vi "Make_PS_Req.vi"(8 "error in (no error)":errorcluster, 11 "Request in":refnum<class "Request.lvclass">) -> (0 "error out":errorcluster, 1 "standard error":string, 2 "standard output":string, 3 "Request out":refnum<class "Request.lvclass">)   [LabVIEW 2016, in "Request.lvclass"]
uses:
  Request.lvclass
  Request.lvclass/Request.ctl
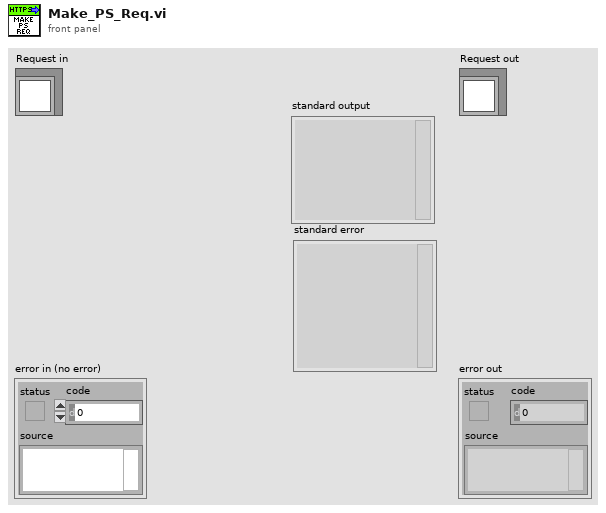
[diagram p1: front panel]
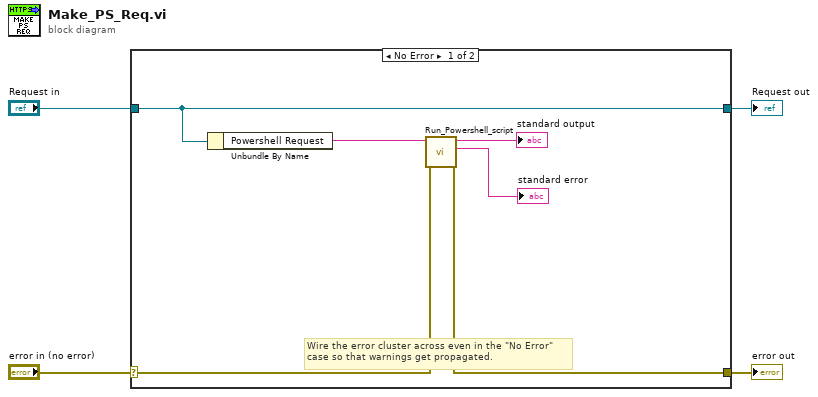
[diagram p0: block diagram]
diagram:
  n1 = case shown="No Error" "error in (no error)" {
    selector: "error in (no error)" -> [w8 w12]
    tunnel: [w7 w12] -> w3
    tunnel: [w10 w11] -> w1
    tunnel: "Request in" -> [w10 w11]
    frame No Error {
      # "Wire the error cluster across even in the \"No Error\"\ncase so that warnings get propagated."
      n2 = Unbundle By Name(w10) -> ("Powershell Request"=w9:string)
      n3 = call "Run_Powershell_script.vi"("error in"=w8, "Powershell Script"=w9) -> ("error out"=w7:errorcluster, "standard error"=→"standard error":string, "standard output"=→"standard output":string)  [unwired: 7 in]
    }
    frame Error {
    }
  }
  "error out" <- w3
  "Request out" <- w1
